vi "Get Rabi Params.vi"(11 "Rabi Parameters":T1={"Window 1 time (s)"=3e-06, "Window 2 time (s)"=5e-06, "Window 3 min time (s) "=0.0, "Window 3 max time (s)"=0.0, "Window 4 time (s)"=7.5e-07, "Window 5 time (s)"=2e-07, "Window 6 time (s)"=3e-06, "Window 7 time (s)"=2e-07, "Window 8 time (s)"=1e-07, "# samples before track"=0, "# time axis points"=0, "Window 1 active channels"=[FALSE, FALSE, FALSE, TRUE], "Window 2 active channels"=[], "Window 3 active channels"=[TRUE], "Window 4 active channels"=[FALSE, FALSE, FALSE, TRUE], "Window 5 active channels "=[FALSE, FALSE, TRUE, TRUE], "Window 6 active channels"=[FALSE, FALSE, FALSE, TRUE], "Window 7 active channels"=[FALSE, FALSE, TRUE, TRUE], "Window 8 active channels"=[], "Path to Rabi Burner"=path "C:/Users/Loncar/Desktop/ESR VIs - Srujan/Sam Kim/PB/RabiBurn.exe"}) -> (0 "max time":dbl, 1 "min time":dbl, 2 "# time points":i32, 3 "# samples":i32, 4 "PB Window Args":string)   [LabVIEW 2012]
uses:
  Rabi Window Parameters.ctl
panel:
  # "Initialization"
  # "Green AOM"
  # "Wait"
  # "All off"
  # "MW pulsing"
  # "MW"
  # "Wait"
  # "Green AOM"
  # "Green AOM,\ncounter sample clk"
  # "Readout"
  # "Repump"
  # "Green AOM"
  # "Green AOM,\ncounter sample clk"
  # "Reference"
  # "All off"
  # "Wait (nominal)"
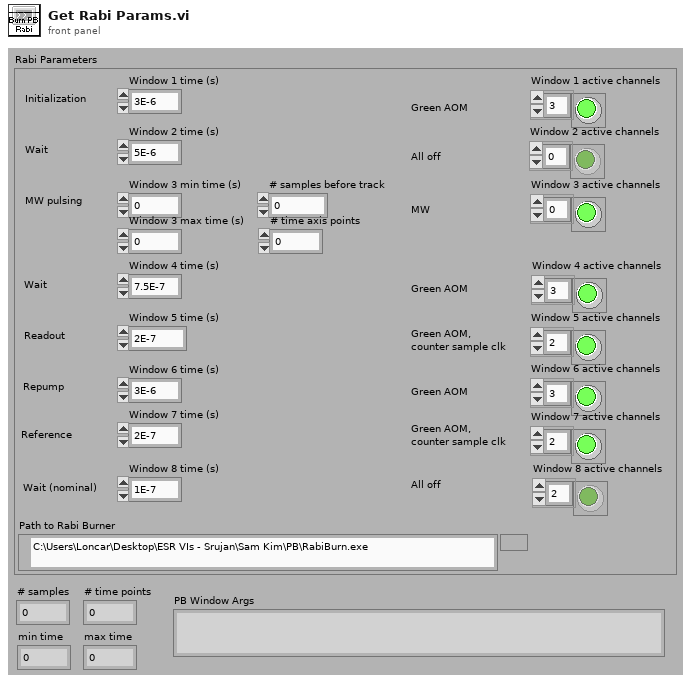
[diagram p1: front panel]
types:
  T1 = typedef "Rabi Window Parameters.ctl" = cluster{"Window 1 time (s)":dbl, "Window 2 time (s)":dbl, "Window 3 min time (s) ":dbl, "Window 3 max time (s)":dbl, "Window 4 time (s)":dbl, "Window 5 time (s)":dbl, "Window 6 time (s)":dbl, "Window 7 time (s)":dbl, "Window 8 time (s)":dbl, "# samples before track":i32, "# time axis points":i32, "Window 1 active channels":bool[], "Window 2 active channels":bool[], "Window 3 active channels":bool[], "Window 4 active channels":bool[], "Window 5 active channels ":bool[], "Window 6 active channels":bool[], "Window 7 active channels":bool[], "Window 8 active channels":bool[], "Path to Rabi Burner":path}
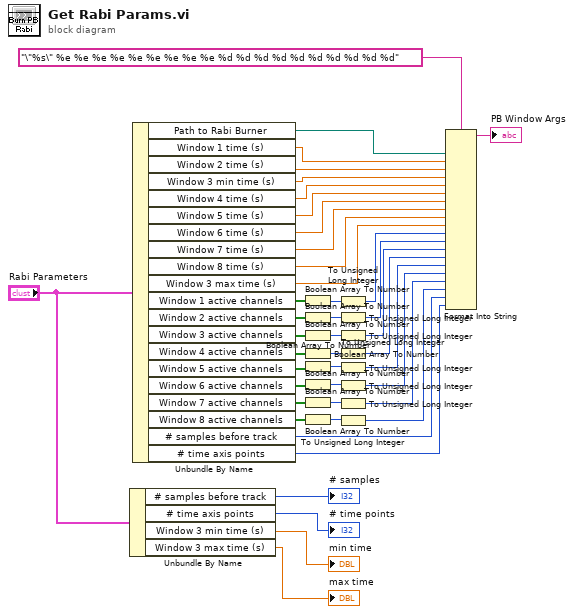
[diagram p0: block diagram]
diagram:
  n1 = Unbundle By Name("Rabi Parameters") -> ("# samples before track"=→"# samples":i32, "# time axis points"=→"# time points":i32, "Window 3 min time (s)"=→"min time":dbl, "Window 3 max time (s)"=→"max time":dbl)
  n2 = Unbundle By Name("Rabi Parameters") -> ("Path to Rabi Burner"=w34:path, "Window 1 time (s)"=w38:dbl, "Window 2 time (s)"=w37:dbl, "Window 3 min time (s)"=w36:dbl, "Window 4 time (s)"=w35:dbl, "Window 5 time (s)"=w33:dbl, "Window 6 time (s)"=w32:dbl, "Window 7 time (s)"=w31:dbl, "Window 8 time (s)"=w30:dbl, "Window 3 max time (s)"=w29:dbl, "Window 1 active channels"=w28:bool[], "Window 2 active channels"=w27:bool[], "Window 3 active channels"=w26:bool[], "Window 4 active channels"=w25:bool[], "Window 5 active channels"=w20:bool[], "Window 6 active channels"=w19:bool[], "Window 7 active channels"=w18:bool[], "Window 8 active channels"=w17:bool[], "# samples before track"=w8:i32, "# time axis points"=w7:i32)
  n3 = Boolean Array To Number(Boolean array=w28) -> (number=w42:u32)
  n4 = Boolean Array To Number(Boolean array=w27) -> (number=w41:u32)
  n5 = Boolean Array To Number(Boolean array=w26) -> (number=w40:u32)
  n6 = Boolean Array To Number(Boolean array=w25) -> (number=w39:u32)
  n7 = Boolean Array To Number(Boolean array=w20) -> (number=w24:u32)
  n8 = Boolean Array To Number(Boolean array=w19) -> (number=w23:u32)
  n9 = Boolean Array To Number(Boolean array=w18) -> (number=w22:u32)
  n10 = Boolean Array To Number(Boolean array=w17) -> (number=w21:u32)
  n11 = To Unsigned Long Integer(number=w42) -> (unsigned 32bit integer=w16:u32)
  n12 = To Unsigned Long Integer(number=w41) -> (unsigned 32bit integer=w15:u32)
  n13 = To Unsigned Long Integer(number=w40) -> (unsigned 32bit integer=w14:u32)
  n14 = To Unsigned Long Integer(number=w39) -> (unsigned 32bit integer=w13:u32)
  n15 = To Unsigned Long Integer(number=w24) -> (unsigned 32bit integer=w12:u32)
  n16 = To Unsigned Long Integer(number=w23) -> (unsigned 32bit integer=w11:u32)
  n17 = To Unsigned Long Integer(number=w22) -> (unsigned 32bit integer=w10:u32)
  n18 = To Unsigned Long Integer(number=w21) -> (unsigned 32bit integer=w9:u32)
  n19 = Format Into String(format string="\"%s\" %e %e %e %e %e %e %e %e %e %d %d %d %d %d %d %d %d %d %d", w34, w38, w37, w36, w35, w33, w32, w31, w30, w29, w16, w15, w14, w13, w12, w11, w10, w9, w8, w7) -> (resulting string=→"PB Window Args":string)  [unwired: 2 in, 1 out]
